vi "Load Grid from File.vi"(8 "error in (no error)":errorcluster, 11 "file path":path) -> (0 "error out":errorcluster, 1 "cancelled":bool, 3 "occupancy grid":dbl[][](array[numeric]))   [LabVIEW 2016]
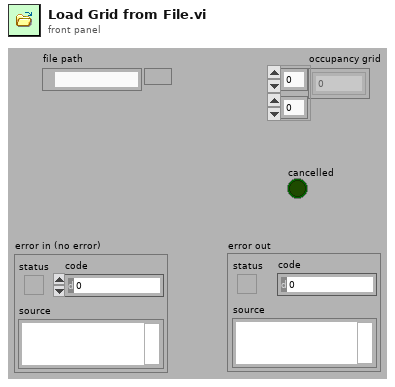
[diagram p1: front panel]
types:
  T1 = enum16{"open", "replace", "create", "open or create", "replace or create", "replace or create with confirmation"}
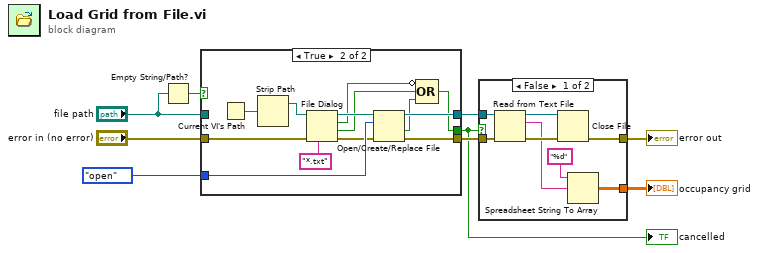
[diagram p0: block diagram]
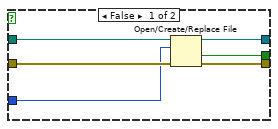
[diagram p3: hidden frame]
diagram:
  n1 = Empty String/Path?(string/path="file path") -> (empty?=w3:bool)
  n2 = case shown="True" w3 {
    tunnel: [w15 w28] -> w9
    tunnel: [w14 w27] -> w8
    tunnel: "error in (no error)" -> [w13 w25]
    tunnel: T1."open" ("operation (0:open)") -> [w12 w26]
    tunnel: "file path" -> [w11 _]
    tunnel: [w10 w19] -> w1
    frame False {
      n3 = Open/Create/Replace File(file path (use dialog)=w11, error in=w13, operation (0:open)=w12) -> (refnum out=w15:refnum<file>, cancelled=w10:bool, error out=w14:errorcluster)  [unwired: 3 in]
    }
    frame True {
      n4 = Current VI's Path() -> (path=w18:path)
      n5 = Strip Path(path=w18) -> (stripped path=w17:path)  [unwired: 1 out]
      n6 = File Dialog(6:"*.txt" ("pattern (all files)"), 8:w25, 11:w17) -> (0:w24:errorcluster, 1:w21:bool, 2:w22:bool, 3:w23:path)  [unwired: 4 in]
      n7 = Open/Create/Replace File(file path (use dialog)=w23, error in=w24, operation (0:open)=w26) -> (refnum out=w28:refnum<file>, cancelled=w20:bool, error out=w27:errorcluster)  [unwired: 3 in]
      n8 = Compound Arithmetic op=OR(invert w22, w21, w20) -> (w19:bool)
    }
  }
  "cancelled" <- w1
  n9 = case shown="False" w1 {
    tunnel: w9 -> [w36 _]
    tunnel: w8 -> [w35 _]
    tunnel: [w32 _] -> w7
    tunnel: [w29 _] -> w2
    frame False {
      n10 = Read from Text File(file (use dialog)=w36, error in=w35) -> (refnum out=w34:refnum<file>, text=w31:string, error out=w33:errorcluster)  [unwired: 2 in, 1 out]
      n11 = Close File(refnum=w34, error in=w33) -> (error out=w32:errorcluster)  [unwired: 1 out]
      n12 = Spreadsheet String To Array(format string="%d", spreadsheet string=w31) -> (array=w29:dbl[][])  [unwired: 2 in]
    }
    frame True {
    }
  }
  "occupancy grid" <- w2
  "error out" <- w7
